vi "Perform Flips.vi"(8 "error in (no error)":errorcluster, 10 "Choice":T1, 11 "Reversi in":refnum<class "Reversi.lvclass">) -> (0 "error out":errorcluster, 3 "Reversi out":refnum<class "Reversi.lvclass">)   [LabVIEW 2020, in "Reversi.lvlib" / "Reversi.lvclass"]
uses:
  Reversi.lvclass
  Space Ring.ctl
  Space Coordinates.ctl
  Space Cluster.ctl
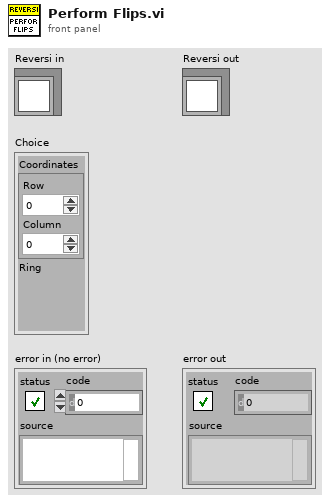
[diagram p1: front panel]
types:
  T1 = typedef "Reversi.lvlib/Reversi.lvclass/Space Cluster.ctl" = cluster{"Coordinates":T2, "Ring":T3}
  T2 = typedef "Reversi.lvlib/Reversi.lvclass/Space Coordinates.ctl" = cluster{"Row":i32, "Column":i32}
  T3 = typedef "Reversi.lvlib/Reversi.lvclass/Space Ring.ctl" = u16
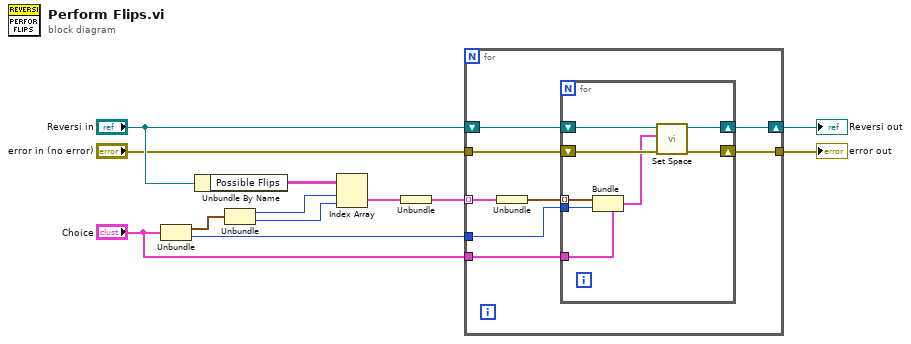
[diagram p0: block diagram]
diagram:
  n1 = Unbundle("Choice") -> ("Coordinates"=w11:T2, "Ring"=w2:T3)
  n2 = Unbundle By Name("Reversi in") -> ("Possible Flips"=w12:cluster{"Possible Flips":cluster{T2[]}[]}[][])
  n3 = Unbundle(w11) -> ("Row"=w10:i32, "Column"=w9:i32)
  n4 = Index Array(array=w12, index (row)=w10, index (col)=w9) -> (element=w8:cluster{"Possible Flips":cluster{T2[]}[]})
  n5 = Unbundle(w8) -> ("Possible Flips"=w5:cluster{T2[]}[])
  n6 = for {
    shift-right: [w19] -> w6
    shift-left: "Reversi in" -> [w20]
    tunnel: w5 -> [w18] mode=indexing
    tunnel: "error in (no error)" -> [w17]
    tunnel: [w16] -> w3
    tunnel: w2 -> [w13]
    tunnel: "Choice" -> [w15]
    n7 = Unbundle(w18) -> (w14:T2[])
    n8 = for {
      tunnel: w15 -> [w24]
      shift-right: [w27] -> w19
      shift-left: w20 -> [w28]
      shift-right: [w25] -> w16
      shift-left: w17 -> [w26]
      tunnel: w14 -> [w23] mode=indexing
      tunnel: w13 -> [w21]
      n9 = Bundle(cluster=w24, "Coordinates"=w23, "Ring"=w21) -> (w22:T1)
      n10 = call "Set Space.vi"("error in (no error)"=w26, "Space"=w22, "Reversi in"=w28) -> ("error out"=w25:errorcluster, "Reversi out"=w27:refnum<class "Reversi.lvclass">)  [unwired: 7 in]
    }
  }
  "error out" <- w3
  "Reversi out" <- w6
